vi "remove channel.vi"(8 "error in (no error)":errorcluster, 10 "channel":refnum<class "TBM channel.lvclass">, 11 "E2E configuration in":refnum<class "E2E Tag Exchange configuration.lvclass">) -> (0 "error out":errorcluster, 2 "removed channel":refnum<class "TBM channel.lvclass">, 3 "E2E configuration out":refnum<class "E2E Tag Exchange configuration.lvclass">)   [LabVIEW 2015, in "E2E Tag Exchange configuration.lvclass"]
uses:
  E2E Tag Exchange configuration.lvclass
  <vilib>/NI/Tag Bus Module Framework/channel/TBM channel.lvclass
  E2E Tag Exchange configuration.lvclass/E2E Tag Exchange configuration.ctl
  <vilib>/NI/Tag Bus/tag/tag descriptor.lvclass/tag descriptor.ctl
  <vilib>/NI/Tag Bus/tag/tag descriptor.lvclass
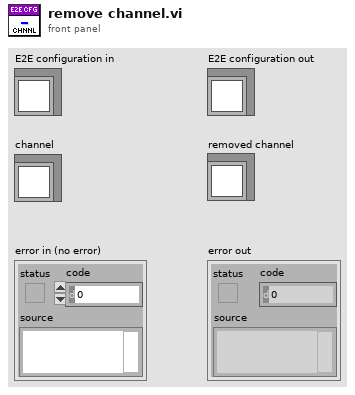
[diagram p1: front panel]
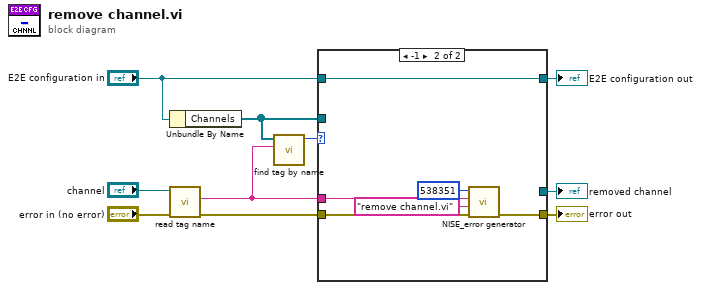
[diagram p0: block diagram]
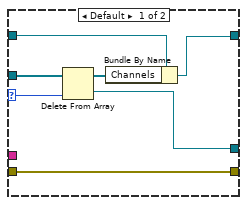
[diagram p2: hidden frame]
diagram:
  n1 = Unbundle By Name("E2E configuration in") -> ("Channels"=w7:refnum<class "TBM channel.lvclass">[])
  n2 = call <vilib>:"read tag name.vi"("error in"="error in (no error)", "system tag in"="channel") -> ("error out"=w5:errorcluster, "name"=w1:string)  [unwired: 7 in, 1 out]
  n3 = call <vilib>:"find tag by name.vi"("name"=w1, "tags in"=w7) -> ("index"=w9:i32)  [unwired: 9 in]
  n4 = case shown="-1" w9 {
    selector: w9 -> [w12 _]
    tunnel: "E2E configuration in" -> [w17 w23]
    tunnel: w7 -> [w16 _]
    tunnel: w5 -> [w15 w22]
    tunnel: [w15 w21] -> w4
    tunnel: [w14 w23] -> w3
    tunnel: [w11 _] -> w2
    tunnel: w1 -> [_ w18]
    frame Default {
      n5 = Delete From Array(array=w16, index=w12) -> (deleted portion=w11:refnum<class "TBM channel.lvclass">, array with subset deleted=w13:refnum<class "TBM channel.lvclass">[])  [unwired: 1 in]
      n6 = Bundle By Name(cluster=w17, "Channels"=w13) -> (w14:refnum<class "E2E Tag Exchange configuration.lvclass">)
    }
    frame -1 {
      n7 = call <vilib>:"NISE_error generator.vi"("error in"=w22, "source"="remove channel.vi", "append error message"=w18, "error code (0)"=538351) -> ("error out"=w21:errorcluster)  [unwired: 5 in]
    }
  }
  "error out" <- w4
  "E2E configuration out" <- w3
  "removed channel" <- w2
